vi "Validate RT Address.vi"(4 "RT Address (0-30)":u8, 6 "RT 1?":bool, 8 "error in (no error)":errorcluster, 11 "Remote Terminal in":refnum<class "Remote Terminal.lvclass">) -> (0 "error out":errorcluster, 3 "Remote Terminal out":refnum<class "Remote Terminal.lvclass">)   [LabVIEW 2020, in "Unit Tests.lvlib" / "Remote Terminal.lvclass"]
uses:
  Remote Terminal.lvclass
  Remote Terminal.lvclass/Remote Terminal.ctl
  <vilib>/addons/_JKI Toolkits/Caraya/classes/Assert/Assert True.vi
  Dependencies/FPGA Interface/FPGA Interface.lvclass
  <vilib>/addons/_JKI Toolkits/Caraya/classes/Test/Test.lvclass
  <vilib>/addons/_JKI Toolkits/Caraya/classes/Assert/Assert.lvclass
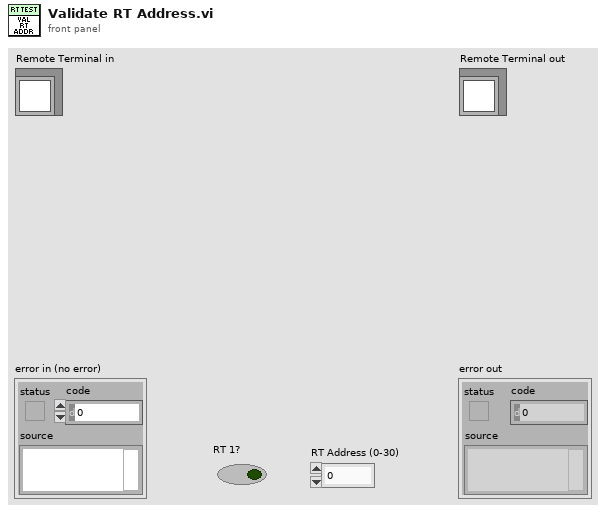
[diagram p1: front panel]
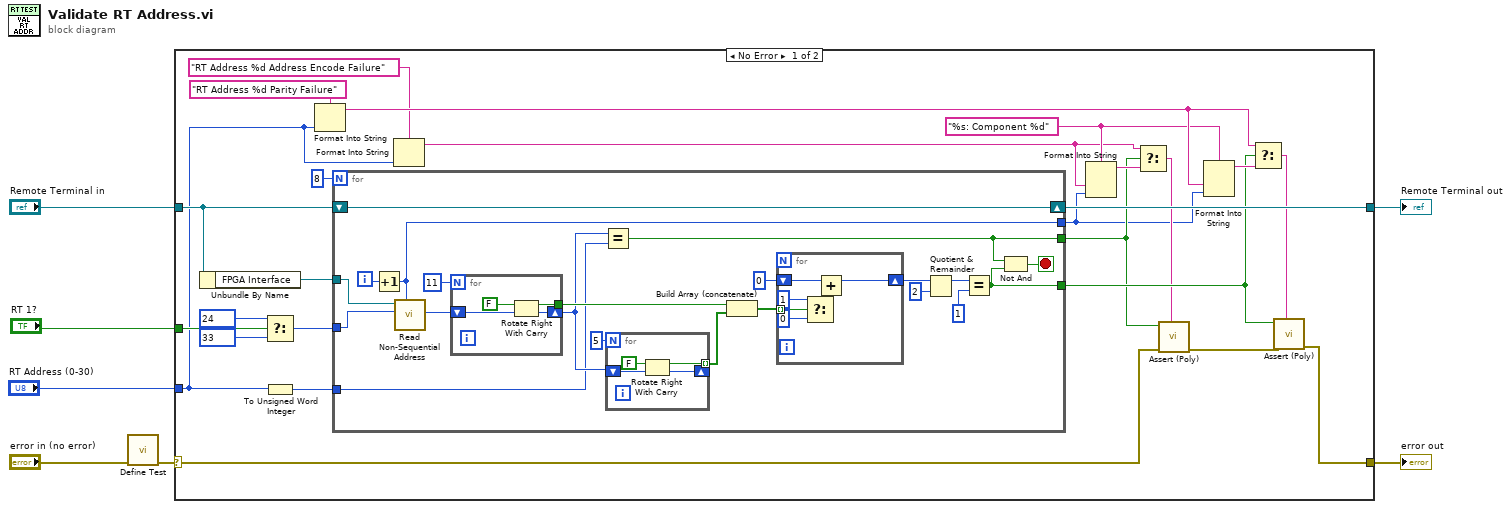
[diagram p0: block diagram]
diagram:
  n1 = call <vilib>:"Define Test.vi"("error in (no error)"="error in (no error)") -> ("error out"=w3:errorcluster)  [unwired: 9 in, 1 out]
  n2 = case shown="No Error" w3 {
    selector: w3 -> [w9 w69]
    tunnel: [w8 w69] -> w2
    tunnel: [w27 w68] -> w6
    tunnel: "Remote Terminal in" -> [w29 w68]
    tunnel: "RT 1?" -> [w30 _]
    tunnel: "RT Address (0-30)" -> [w13 _]
    frame No Error {
      w18 = "%s: Component %d"
      n3 = Unbundle By Name(w29) -> ("FPGA Interface"=w26:refnum<class "FPGA Interface.lvclass">)
      n4 = Select(t=u16 24, s=w30, f=u16 33) -> (s? t:f=w25:u16)
      n5 = To Unsigned Word Integer(number=w13) -> (unsigned 16bit integer=w24:u16)
      n6 = Format Into String(format string="RT Address %d Parity Failure", w13) -> (resulting string=w21:string)  [unwired: 2 in, 1 out]
      n7 = for {
        N: 8 -> [_]
        shift-right: [w41] -> w27
        shift-left: w29 -> [w41]
        tunnel: w26 -> [w53]
        tunnel: w25 -> [w51]
        tunnel: w24 -> [w37]
        tunnel: [w36] -> w20
        tunnel: [w35] -> w16
        tunnel: [w33] -> w14
        i -> [w52]
        stop <- w34 stop-if-true
        n8 = Increment(x=w52) -> (x+1=w33:i32)
        n9 = call-dynamic "Read Non-Sequential Address.vi"("Target IC (1-8)"=w33, "Address"=w51, "FPGA Interface in"=w53) -> ("Data"=w49:u16)  [unwired: 7 in, 1 out]
        n10 = for {
          N: 11 -> [_]
          tunnel: [w66] -> w47
          shift-right: [w65] -> w38
          shift-left: w49 -> [w67]
          n11 = Rotate Right With Carry(2:w67, 3:FALSE ("carry")) -> (0:w65:u16, 1:w66:bool)
        }
        n12 = Equal?(x=w38, y=w37) -> (x = y?=w35:bool)
        n13 = for {
          N: 5 -> [_]
          shift-right: [w62] -> _
          shift-left: w38 -> [w63]
          tunnel: [w61] -> w46 mode=indexing
          n14 = Rotate Right With Carry(2:w63, 3:FALSE ("carry")) -> (0:w62:u16, 1:w61:bool)
        }
        n15 = Build Array (concatenate)(w47, w46) -> (w44:bool[])
        n16 = for {
          tunnel: w44 -> [w57] mode=indexing
          shift-right: [w58] -> w42
          shift-left: 0 -> [w59]
          n17 = Select(t=1, s=w57, f=0) -> (s? t:f=w54:i32)
          n18 = Add(x=w59, y=w54) -> (x+y=w58:i32)
        }
        n19 = Quotient & Remainder(x=w42, y=2) -> (x-y*floor(x/y)=w40:i32)  [unwired: 1 out]
        n20 = Equal?(x=w40, y=1 ("x-y*floor(x/y)")) -> (x = y?=w36:bool)
        n21 = Not And(1:w36, 2:w35) -> (0:w34:bool)
      }
      n22 = Format Into String(format string="RT Address %d Address Encode Failure", w13) -> (resulting string=w11:string)  [unwired: 2 in, 1 out]
      n23 = Format Into String(format string=w18, w11, w14) -> (resulting string=w17:string)  [unwired: 2 in, 1 out]
      n24 = Select(t=w11, s=w16, f=w17) -> (s? t:f=w15:string)
      n25 = call-poly <vilib>:"Assert (Poly).vi"("Label"=w15, "error in (no error)"=w9, "True?"=w16) -> ("error out"=w10:errorcluster)  [unwired: 7 in, 1 out]
      n26 = Format Into String(format string=w18, w21, w14) -> (resulting string=w22:string)  [unwired: 2 in, 1 out]
      n27 = Select(t=w21, s=w20, f=w22) -> (s? t:f=w19:string)
      n28 = call-poly <vilib>:"Assert (Poly).vi"("Label"=w19, "error in (no error)"=w10, "True?"=w20) -> ("error out"=w8:errorcluster)  [unwired: 7 in, 1 out]
    }
    frame Error {
    }
  }
  "error out" <- w2
  "Remote Terminal out" <- w6
